vi "RampVoltagewithDDSv6,rampgenFF.vi"(6 "No of samples in ramp":dbl, 7 "Trigger delay NI (ms)":dbl, 8 "DDS Trigger Delay (ms)":dbl, 9 "Ramp Amplitude (V)}":dbl, 10 "Ramp duration (ms)":dbl, 11 "Plateau duration (ms)":dbl) -> (1 "Numeric 2":i32, 2 "Numeric":dbl, 3 "Sample rate":dbl=500000.0, 4 "Array":dbl[](array[numeric]))   [LabVIEW 2016]
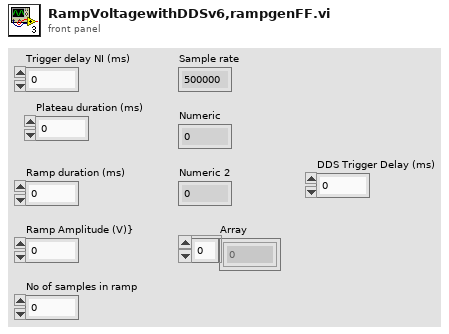
[diagram p1: front panel]
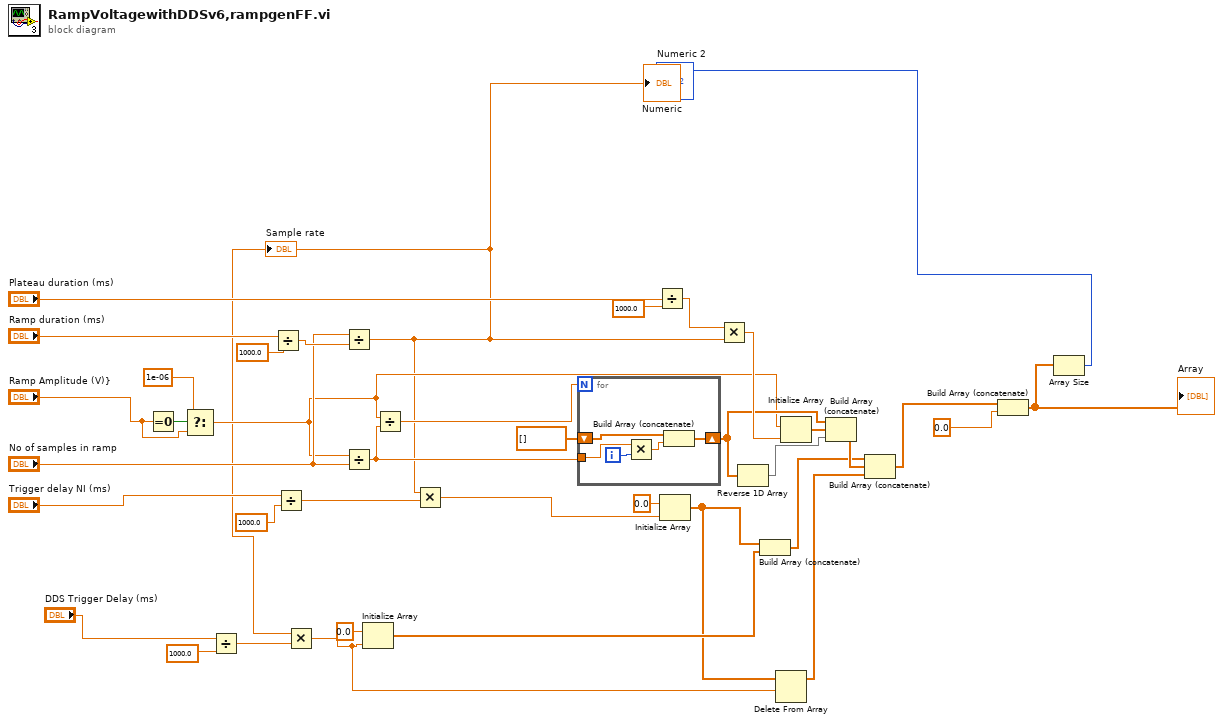
[diagram p0: block diagram]
diagram:
  n1 = Equal To 0?(x="Ramp Amplitude (V)}") -> (x = 0?=w14:bool)
  n2 = Select(t=1e-06, s=w14, f="Ramp Amplitude (V)}") -> (s? t:f=w12:dbl)
  n3 = Divide(x="DDS Trigger Delay (ms)", y=1000.0) -> (x/y=w7:dbl)
  n4 = Divide(x="Ramp duration (ms)", y=1000.0) -> (x/y=w22:dbl)
  n5 = Divide(x="Trigger delay NI (ms)", y=1000.0) -> (x/y=w30:dbl)
  n6 = Divide(x="No of samples in ramp", y=w22) -> (x/y=w8:dbl)
  "Sample rate" <- w8
  "Numeric" <- w8
  n7 = Multiply(x=w8, y=w7) -> (x*y=w5:dbl)
  n8 = Divide(x=w12, y="No of samples in ramp") -> (x/y=w16:dbl)
  n9 = Initialize Array(0.0 ("element"), w5) -> (w4:dbl[])
  n10 = Divide(x=w12, y=w16) -> (x/y=w32:dbl)
  n11 = Multiply(x=w8, y=w30) -> (x*y=w31:dbl)
  n12 = for {
    N: w32 -> [_]
    shift-right: [w41] -> w17
    shift-left: dbl[] [] -> [w40]
    tunnel: w16 -> [w39]
    i -> [w43]
    n13 = Multiply(x=w39, y=w43) -> (x*y=w42:dbl)
    n14 = Build Array (concatenate)(w40, w42) -> (w41:dbl[])
  }
  n15 = Divide(x="Plateau duration (ms)", y=1000.0) -> (x/y=w24:dbl)
  n16 = Initialize Array(0.0 ("element"), w31) -> (w3:dbl[])
  n17 = Multiply(x=w24, y=w8) -> (x*y=w25:dbl)
  n18 = Reverse 1D Array(array=w17) -> (reversed array=w19:dbl[])
  n19 = Build Array (concatenate)(w3, w4) -> (w2:dbl[])
  n20 = Delete From Array(array=w3, length=w5) -> (array with subset deleted=w1:dbl[])  [unwired: 1 in, 1 out]
  n21 = Initialize Array(w12, w25) -> (w18:dbl[])
  n22 = Build Array (concatenate)(w17, w18, w19) -> (w27:dbl[])
  n23 = Build Array (concatenate)(w2, w27, w1) -> (w35:dbl[])
  n24 = Build Array (concatenate)(w35, 0.0 ("y")) -> (w38:dbl[])
  "Array" <- w38
  n25 = Array Size(array=w38) -> (size(s)=→"Numeric 2":i32)
